vi "SetDevice_popup.vi"(2 "Input Line Command":string, 3 "error in (no error)":errorcluster) -> (8 "Cancel":bool, 9 "Output Line Command":string, 10 "error out":errorcluster)   [LabVIEW 2020]
uses:
  Device_List.ctl
  Unit_List.ctl
panel:
  in  "Motor":T1 caption="Unit"
  in  "platform":u16(ring) items=["Mac", "PC"]
  in  "372 unit":T1 caption="Unit"
  in  "372 ch#":T1 caption="Unit"
  in  "370 heater":T1 caption="Unit"
  in  "37X range":T1 caption="Unit"
  in  "37X Iex":T1 caption="Unit"
  in  "370 ch#":T1 caption="Unit"
  out "comment":string
  in  "heater value":T1 caption="Unit"
  in  "sensor value":T1 caption="Unit"
  in  "Cancel Button":bool
  in  "OK Button":bool
  in  "VISA resource name":refnum<visa-resource-name>
  in  "Unit":T1
  in  "Value":string="0"
  in  "Device":T2
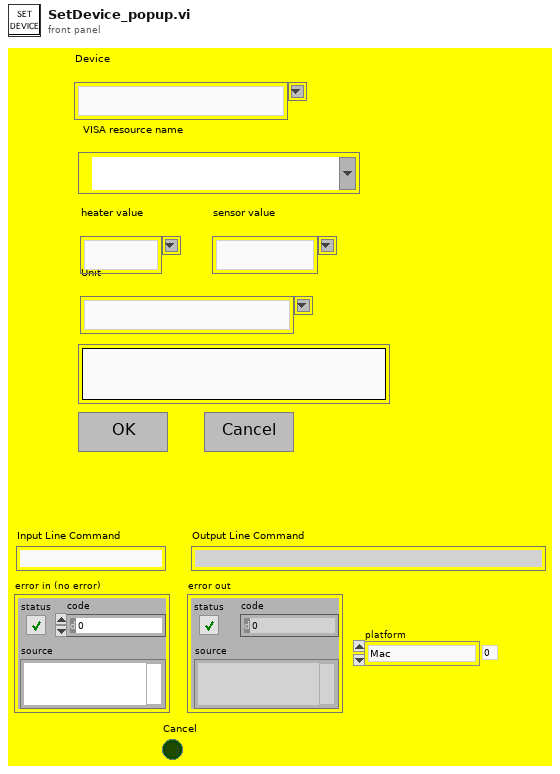
[diagram p1: front panel]
types:
  T1 = typedef "Unit_List.ctl" = string
  T2 = typedef "Device_List.ctl" = string
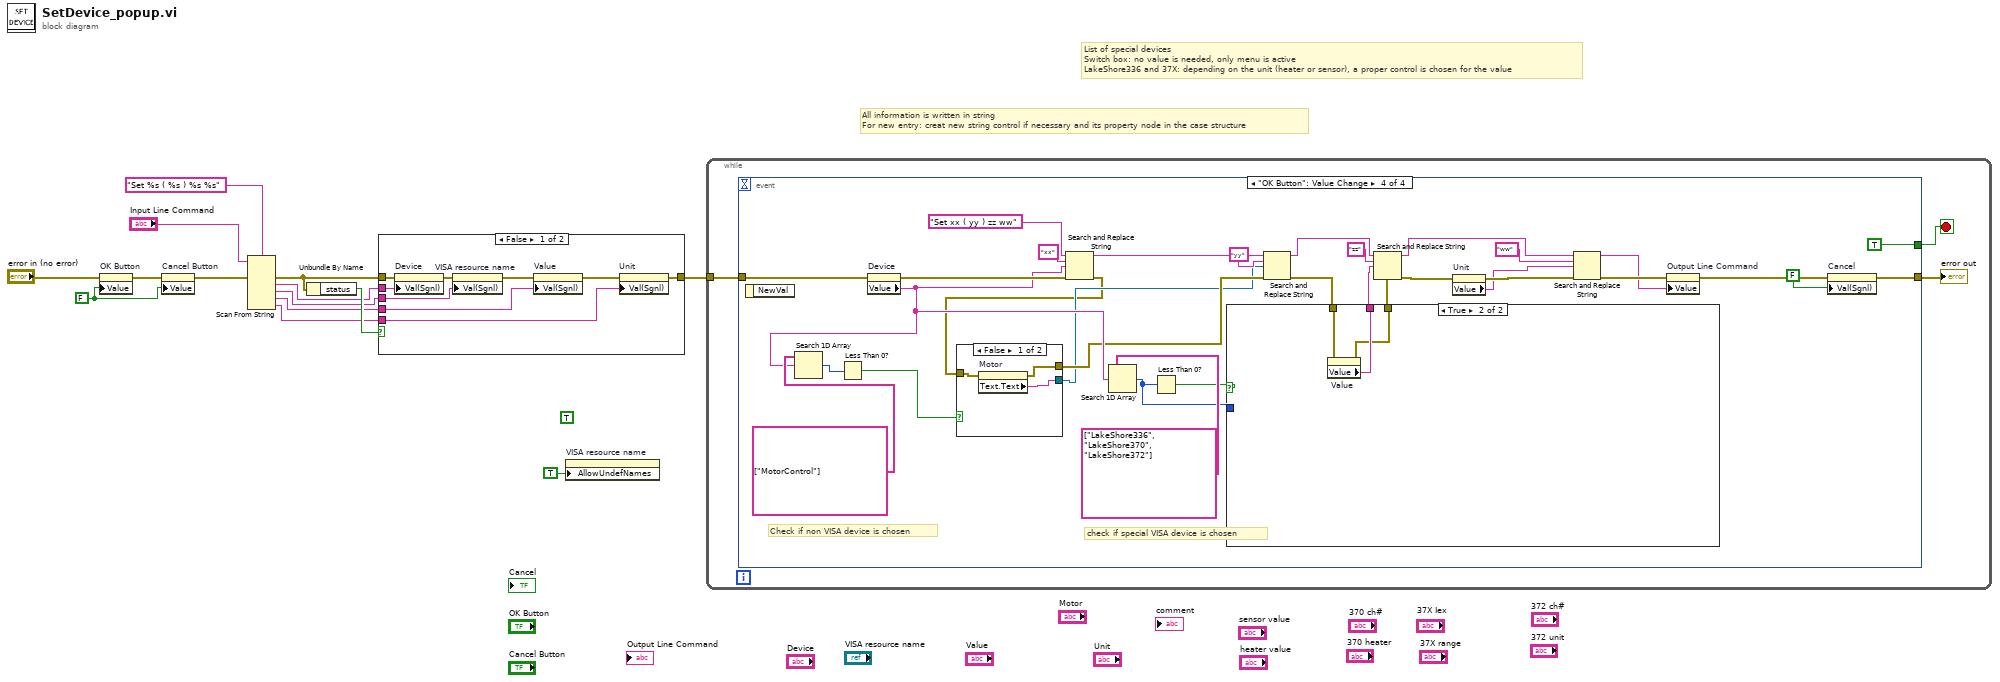
[diagram p0: block diagram]
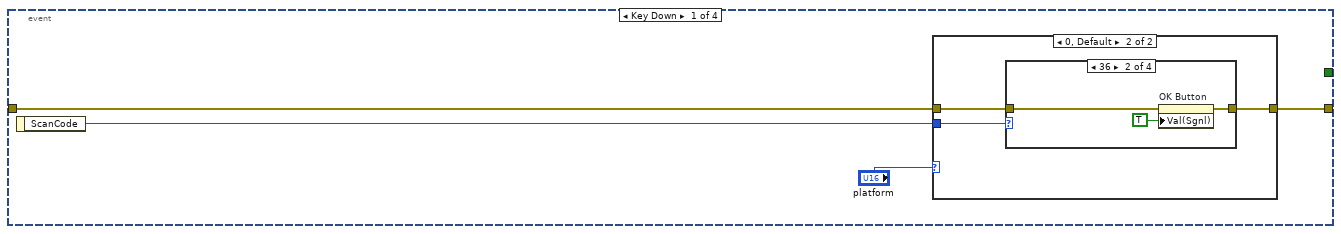
[diagram p2: hidden frame]
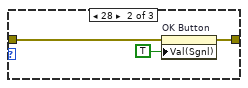
[diagram p4: hidden frame]
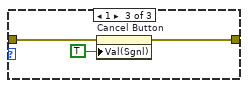
[diagram p5: hidden frame]
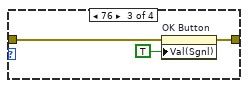
[diagram p7: hidden frame]
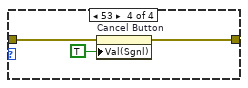
[diagram p8: hidden frame]
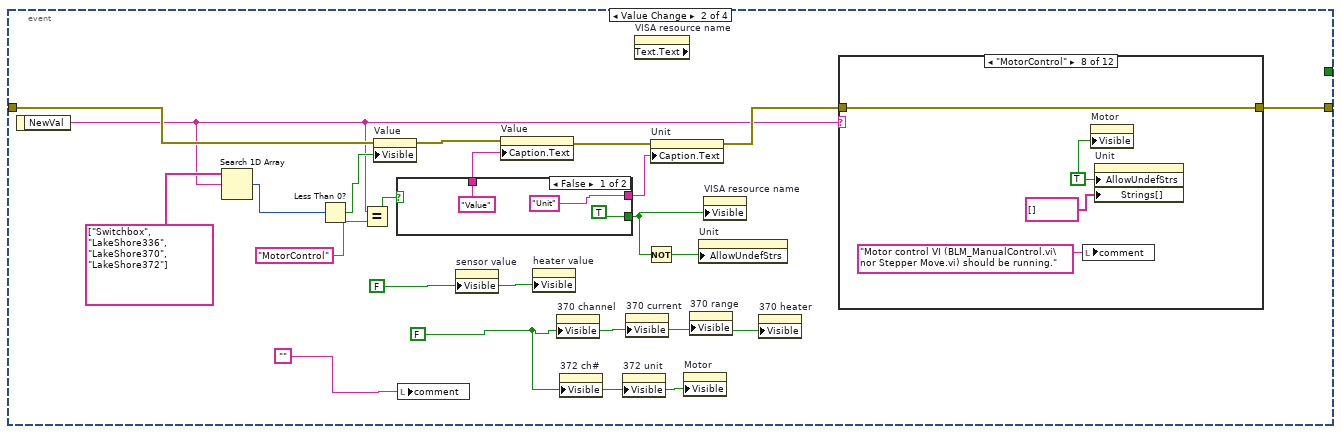
[diagram p9: hidden frame]
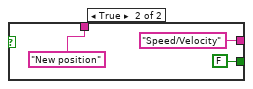
[diagram p10: hidden frame]
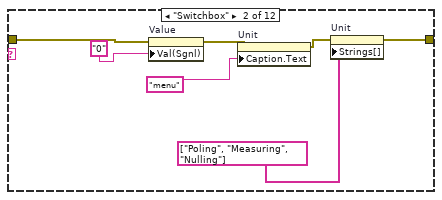
[diagram p12: hidden frame]
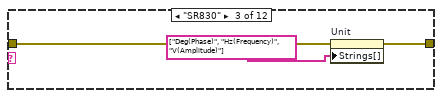
[diagram p13: hidden frame]
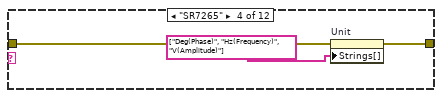
[diagram p14: hidden frame]
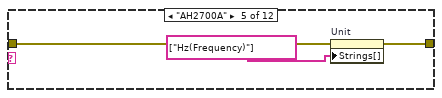
[diagram p15: hidden frame]
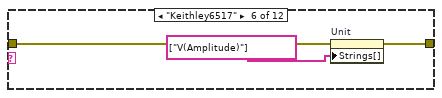
[diagram p16: hidden frame]
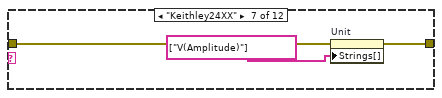
[diagram p17: hidden frame]
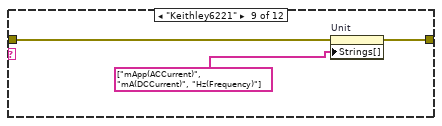
[diagram p18: hidden frame]
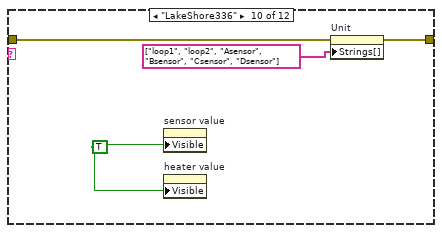
[diagram p19: hidden frame]
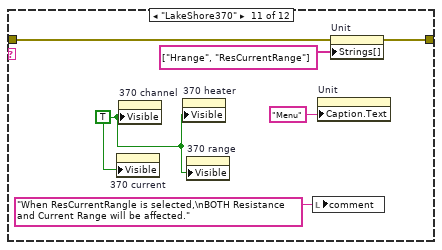
[diagram p20: hidden frame]
diagram:
  (unwired) TRUE ("Visible")
  w12 = FALSE
  # "List of special devices\nSwitch box: no value is needed, only menu is active\nLakeShore336 and 37X: depending on the unit (heater or sensor), a proper control is chosen for the value"
  # "All information is written in string\nFor new entry: creat new string control if necessary and its property node in the case structure"
  n1 = property on="OK Button" class="Bool (strict)"(error in="error in (no error)", "Value"=w12) -> (error out=w13:errorcluster)  [unwired: 1 in, 1 out]
  n2 = property on="Cancel Button" class="Bool (strict)"(error in=w13, "Value"=w12) -> (error out=w11:errorcluster)  [unwired: 1 in, 1 out]
  n3 = Scan From String(format string="Set %s ( %s ) %s %s", input string="Input Line Command", error in=w11) -> (error out=w7:errorcluster, output 1=w6:string, output 2=w5:string, output 3=w4:string, output 4=w3:string)  [unwired: 5 in, 2 out]
  n4 = Unbundle By Name(w7) -> ("status"=w8:bool)
  n5 = case shown="False" w8 {
    tunnel: w7 -> [w23 w25]
    tunnel: [w15 w24] -> w2
    tunnel: w6 -> [w22 _]
    tunnel: w5 -> [w20 _]
    tunnel: w4 -> [w18 _]
    tunnel: w3 -> [w16 _]
    frame False {
      n6 = property on="Device" class="CmbBox (strict)"(error in=w23, "Val(Sgnl)"=w22) -> (error out=w21:errorcluster)  [unwired: 1 in, 1 out]
      n7 = property on="VISA resource name" class="VISAName"(error in=w21, "Val(Sgnl)"=w20) -> (error out=w19:errorcluster)  [unwired: 1 in, 1 out]
      n8 = property on="Value" class="Str"(error in=w19, "Val(Sgnl)"=w18) -> (error out=w17:errorcluster)  [unwired: 1 in, 1 out]
      n9 = property on="Unit" class="CmbBox (strict)"(error in=w17, "Val(Sgnl)"=w16) -> (error out=w15:errorcluster)  [unwired: 1 in, 1 out]
    }
    frame True {
      n10 = call <vilib>:"Clear Errors.vi"("error in (no error)"=w25) -> ("error out"=w24:errorcluster)  [unwired: 5 in, 1 out]
    }
  }
  n11 = property on="VISA resource name" class="VISAName"("AllowUndefNames"=TRUE ("Allow Undefined Names")) -> ()  [unwired: 2 in, 2 out]
  n12 = while {
    tunnel: w2 -> [w28]
    stop <- w27 stop-if-true
    n13 = event shown="[3] \"OK Button\": Value Change" {
      selector: _ -> [_ _ _ _]
      dyn-events: _ -> [_ _ _ _]
      timeout: _ -> [_ _ _ _]
      tunnel: w28 -> [w31 w72 w127 w157]
      tunnel: [_ _ w126 TRUE ("NewVal")] -> w27
      tunnel: [w30 w73 _ w139] -> w26
      event Key Down {
        n14 = event-data() -> ("ScanCode"=w32:i16)  [unwired: 1 in]
        n15 = case shown="0, Default" "platform" {
          tunnel: w32 -> [w35 w45]
          tunnel: w31 -> [w34 w44]
          tunnel: [w33 w43] -> w30
          frame 1 {
            n16 = case shown="Default" w35 {
              tunnel: w34 -> [w36 w39 w42]
              tunnel: [w36 w37 w40] -> w33
              frame Default {
              }
              frame 28 {
                n17 = property on="OK Button" class="Bool (strict)"(error in=w39, "Val(Sgnl)"=TRUE) -> (error out=w37:errorcluster)  [unwired: 1 in, 1 out]
              }
              frame 1 {
                n18 = property on="Cancel Button" class="Bool (strict)"(error in=w42, "Val(Sgnl)"=TRUE ("Value (Signaling)")) -> (error out=w40:errorcluster)  [unwired: 1 in, 1 out]
              }
            }
          }
          frame 0, Default {
            n19 = case shown="36" w45 {
              tunnel: w44 -> [w46 w49 w52 w55]
              tunnel: [w46 w47 w50 w53] -> w43
              frame Default {
              }
              frame 36 {
                n20 = property on="OK Button" class="Bool (strict)"(error in=w49, "Val(Sgnl)"=TRUE) -> (error out=w47:errorcluster)  [unwired: 1 in, 1 out]
              }
              frame 76 {
                n21 = property on="OK Button" class="Bool (strict)"(error in=w52, "Val(Sgnl)"=TRUE) -> (error out=w50:errorcluster)  [unwired: 1 in, 1 out]
              }
              frame 53 {
                n22 = property on="Cancel Button" class="Bool (strict)"(error in=w55, "Val(Sgnl)"=TRUE ("Value (Signaling)")) -> (error out=w53:errorcluster)  [unwired: 1 in, 1 out]
              }
            }
          }
        }
      }
      event Value Change {
        w57 = FALSE ("Visible")
        w64 = FALSE ("Visible")
        n23 = event-data() -> ("NewVal"=w60:T2)  [unwired: 1 in]
        n24 = Search 1D Array(1D array=string[] ["Switchbox", "LakeShore336", "LakeShore370", "LakeShore372"], element=w60) -> (index of element=w70:i32)  [unwired: 1 in]
        n25 = Less Than 0?(x=w70) -> (x < 0?=w69:bool)
        n26 = Equal?(x=w60, y="MotorControl") -> (x = y?=w59:bool)
        n27 = property on="Value" class="Str"(error in=w72, "Visible"=w69) -> (error out=w67:errorcluster)  [unwired: 1 in, 1 out]
        n28 = case shown="False" w59 {
          tunnel: ["Value" ("Label.Text") "New position" ("Label.Text")] -> w68
          tunnel: ["Unit" ("Label.Text") "Speed/Velocity" ("Label.Text")] -> w62
          tunnel: [TRUE ("Visible") FALSE ("Visible")] -> w56
          frame False {
          }
          frame True {
          }
        }
        n29 = local write "comment"("") -> ()
        n30 = property on="sensor value" class="CmbBox (strict)"("Visible"=w64) -> ()  [unwired: 2 in, 2 out]
        n31 = property on="Value" class="Str"(error in=w67, "Caption.Text"=w68) -> (error out=w66:errorcluster)  [unwired: 1 in, 1 out]
        n32 = property on="heater value" class="CmbBox (strict)"("Visible"=w64) -> ()  [unwired: 2 in, 2 out]
        n33 = property on="370 channel" class="CmbBox (strict)"("Visible"=w57) -> ()  [unwired: 2 in, 2 out]
        n34 = property on="372 ch#" class="CmbBox (strict)"("Visible"=w57) -> ()  [unwired: 2 in, 2 out]
        n35 = property on="372 unit" class="CmbBox (strict)"("Visible"=w57) -> ()  [unwired: 2 in, 2 out]
        n36 = property on="370 current" class="CmbBox (strict)"("Visible"=w57) -> ()  [unwired: 2 in, 2 out]
        n37 = property on="VISA resource name" class="VISAName" props=["Text", "Text"]() -> ()  [unwired: 2 in, 3 out]
        n38 = Not(x=w56) -> (.not. x?=w58:bool)
        n39 = property on="Unit" class="CmbBox (strict)"(error in=w66, "Caption.Text"=w62) -> (error out=w65:errorcluster)  [unwired: 1 in, 1 out]
        n40 = property on="Motor" class="CmbBox (strict)"("Visible"=w57) -> ()  [unwired: 2 in, 2 out]
        n41 = property on="370 range" class="CmbBox (strict)"("Visible"=w57) -> ()  [unwired: 2 in, 2 out]
        n42 = property on="Unit" class="CmbBox (strict)"("AllowUndefStrs"=w58) -> ()  [unwired: 2 in, 2 out]
        n43 = property on="VISA resource name" class="VISAName"("Visible"=w56) -> ()  [unwired: 2 in, 2 out]
        n44 = property on="370 heater" class="CmbBox (strict)"("Visible"=w57) -> ()  [unwired: 2 in, 2 out]
        n45 = case shown="\"MotorControl\"" w60 {
          tunnel: w65 -> [w80 w87 w88 w91 w94 w97 w100 w106 w107 w111 w118 w124]
          tunnel: [w80 w85 w90 w93 w96 w99 w102 w106 w109 w113 w119 w125] -> w73
          frame "False", Default {
          }
          frame "Switchbox" {
            n46 = property on="Value" class="Str"(error in=w87, "Val(Sgnl)"="0" ("Value (Signaling)")) -> (error out=w83:errorcluster)  [unwired: 1 in, 1 out]
            n47 = property on="Unit" class="CmbBox (strict)"(error in=w83, "Caption.Text"="menu") -> (error out=w82:errorcluster)  [unwired: 1 in, 1 out]
            n48 = property on="Unit" class="CmbBox (strict)"(error in=w82, "Strings[]"=string[] ["Poling", "Measuring", "Nulling"] ("Strings []")) -> (error out=w85:errorcluster)  [unwired: 1 in, 1 out]
          }
          frame "SR830" {
            n49 = property on="Unit" class="CmbBox (strict)"(error in=w88, "Strings[]"=string[] ["Deg(Phase)", "Hz(Frequency)", "V(Amplitude)"] ("Strings []")) -> (error out=w90:errorcluster)  [unwired: 1 in, 1 out]
          }
          frame "SR7265" {
            n50 = property on="Unit" class="CmbBox (strict)"(error in=w91, "Strings[]"=string[] ["Deg(Phase)", "Hz(Frequency)", "V(Amplitude)"] ("Strings []")) -> (error out=w93:errorcluster)  [unwired: 1 in, 1 out]
          }
          frame "AH2700A" {
            n51 = property on="Unit" class="CmbBox (strict)"(error in=w94, "Strings[]"=string[] ["Hz(Frequency)"] ("Strings []")) -> (error out=w96:errorcluster)  [unwired: 1 in, 1 out]
          }
          frame "Keithley6517" {
            n52 = property on="Unit" class="CmbBox (strict)"(error in=w97, "Strings[]"=string[] ["V(Amplitude)"] ("Strings []")) -> (error out=w99:errorcluster)  [unwired: 1 in, 1 out]
          }
          frame "Keithley24XX" {
            n53 = property on="Unit" class="CmbBox (strict)"(error in=w100, "Strings[]"=string[] ["V(Amplitude)"] ("Strings []")) -> (error out=w102:errorcluster)  [unwired: 1 in, 1 out]
          }
          frame "MotorControl" {
            w103 = TRUE ("Allow Undefined Strings")
            n54 = local write "comment"("Motor control VI (BLM_ManualControl.vi\nor Stepper Move.vi) should be running." ("comment")) -> ()
            n55 = property on="Motor" class="CmbBox (strict)"("Visible"=w103) -> ()  [unwired: 2 in, 2 out]
            n56 = property on="Unit" class="CmbBox (strict)"("AllowUndefStrs"=w103, "Strings[]"=string[] [] ("Strings []")) -> ()  [unwired: 2 in, 2 out]
          }
          frame "Keithley6221" {
            n57 = property on="Unit" class="CmbBox (strict)"(error in=w107, "Strings[]"=string[] ["mApp(ACCurrent)", "mA(DCCurrent)", "Hz(Frequency)"] ("Strings []")) -> (error out=w109:errorcluster)  [unwired: 1 in, 1 out]
          }
          frame "LakeShore336" {
            w110 = TRUE ("Visible")
            n58 = property on="sensor value" class="CmbBox (strict)"("Visible"=w110) -> ()  [unwired: 2 in, 2 out]
            n59 = property on="heater value" class="CmbBox (strict)"("Visible"=w110) -> ()  [unwired: 2 in, 2 out]
            n60 = property on="Unit" class="CmbBox (strict)"(error in=w111, "Strings[]"=string[] ["loop1", "loop2", "Asensor", "Bsensor", "Csensor", "Dsensor"] ("Strings []")) -> (error out=w113:errorcluster)  [unwired: 1 in, 1 out]
          }
          frame "LakeShore370" {
            w116 = TRUE ("Visible")
            n61 = property on="370 current" class="CmbBox (strict)"("Visible"=w116) -> ()  [unwired: 2 in, 2 out]
            n62 = property on="370 channel" class="CmbBox (strict)"("Visible"=w116) -> ()  [unwired: 2 in, 2 out]
            n63 = property on="370 heater" class="CmbBox (strict)"("Visible"=w116) -> ()  [unwired: 2 in, 2 out]
            n64 = property on="370 range" class="CmbBox (strict)"("Visible"=w116) -> ()  [unwired: 2 in, 2 out]
            n65 = local write "comment"("When ResCurrentRangle is selected,\nBOTH Resistance and Current Range will be affected." ("comment")) -> ()
            n66 = property on="Unit" class="CmbBox (strict)"("Caption.Text"="Menu") -> ()  [unwired: 2 in, 2 out]
            n67 = property on="Unit" class="CmbBox (strict)"(error in=w118, "Strings[]"=string[] ["Hrange", "ResCurrentRange"] ("Strings []")) -> (error out=w119:errorcluster)  [unwired: 1 in, 1 out]
          }
          frame "LakeShore372" {
            w120 = TRUE ("Visible")
            n68 = property on="370 current" class="CmbBox (strict)"("Visible"=w120) -> ()  [unwired: 2 in, 2 out]
            n69 = property on="372 ch#" class="CmbBox (strict)"("Visible"=w120) -> ()  [unwired: 2 in, 2 out]
            n70 = property on="370 range" class="CmbBox (strict)"("Visible"=w120) -> ()  [unwired: 2 in, 2 out]
            n71 = property on="372 unit" class="CmbBox (strict)"("Visible"=w120) -> ()  [unwired: 2 in, 2 out]
            n72 = property on="Unit" class="CmbBox (strict)"("Caption.Text"="Menu") -> ()  [unwired: 2 in, 2 out]
            n73 = property on="Unit" class="CmbBox (strict)"(error in=w124, "Strings[]"=string[] ["ResCurrentRange"] ("Strings []")) -> (error out=w125:errorcluster)  [unwired: 1 in, 1 out]
            n74 = local write "comment"("When ResCurrentRangle is selected,\nAll parameters (Resistance, Current Range, unit) will be affected." ("comment")) -> ()
          }
        }
      }
      event "Cancel Button": Value Change {
        n75 = event-data() -> ("NewVal"=w126:bool)  [unwired: 1 in]
        n76 = property on="Cancel" class="Bool (strict)"(error in=w127, "Value"=w126) -> ()  [unwired: 1 in, 2 out]
      }
      event "OK Button": Value Change {
        # "Check if non VISA device is chosen"
        # "check if special VISA device is chosen"
        n77 = event-data() -> ()  [unwired: 1 in, 1 out]
        n78 = property on="Device" class="CmbBox (strict)"(error in=w157) -> (error out=w156:errorcluster, "Value"=w131:T2)  [unwired: 1 in, 1 out]
        n79 = Search 1D Array(1D array=string[] ["MotorControl"], element=w131) -> (index of element=w134:i32)  [unwired: 1 in]
        n80 = Less Than 0?(x=w134) -> (x < 0?=w133:bool)
        n81 = Search and Replace String(input string="Set xx ( yy ) zz ww", search string="xx", replace string=w131, error in=w156) -> (result string=w154:string, error out=w128:errorcluster)  [unwired: 4 in, 2 out]
        n82 = case shown="False" w133 {
          tunnel: [w161 w165] -> w130
          tunnel: [w160 w164] -> w129
          tunnel: w128 -> [w162 w163]
          frame False {
            n83 = property on="Motor" class="CmbBox (strict)"(error in=w162) -> (error out=w161:errorcluster, "Text.Text"=w160:string)  [unwired: 1 in, 1 out]
          }
          frame True {
            n84 = property on="VISA resource name" class="VISAName"(error in=w163) -> (error out=w165:errorcluster, "Value"=w164:refnum<visa-resource-name>)  [unwired: 1 in, 1 out]
          }
        }
        n85 = Search 1D Array(1D array=string[] ["LakeShore336", "LakeShore370", "LakeShore372"], element=w131) -> (index of element=w135:i32)  [unwired: 1 in]
        n86 = Less Than 0?(x=w135) -> (x < 0?=w136:bool)
        n87 = Search and Replace String(input string=w154, search string="yy", replace string=w129, error in=w130) -> (result string=w153:string, error out=w150:errorcluster)  [unwired: 4 in, 2 out]
        n88 = case shown="True" w136 {
          tunnel: [w166 w222] -> w151
          tunnel: w150 -> [w168 w221]
          tunnel: [w167 w220] -> w149
          tunnel: w135 -> [w169 _]
          frame False {
            n89 = case shown="1" w169 {
              tunnel: w168 -> [w174 w190 w208]
              tunnel: [w173 w189 w207] -> w167
              tunnel: [w172 w184 w203] -> w166
              frame 0, Default {
                # "Lakeshore336"
                n90 = property on="Unit" class="CmbBox (strict)"() -> ("Text.Text"=w170:string)  [unwired: 2 in, 2 out]
                n91 = Match Pattern(string=w170, regular expression="loop") -> (offset past match=w175:i32)  [unwired: 1 in, 3 out]
                n92 = Less Than 0?(x=w175) -> (x < 0?=w171:bool)
                n93 = case shown="False" w171 {
                  tunnel: w174 -> [w179 w182]
                  tunnel: [w178 w181] -> w173
                  tunnel: [w177 w180] -> w172
                  frame False {
                    n94 = property on="heater value" class="CmbBox (strict)"(error in=w179) -> (error out=w178:errorcluster, "Text.Text"=w177:string)  [unwired: 1 in, 1 out]
                  }
                  frame True {
                    n95 = property on="sensor value" class="CmbBox (strict)"(error in=w182) -> (error out=w181:errorcluster, "Text.Text"=w180:string)  [unwired: 1 in, 1 out]
                  }
                }
              }
              frame 1 {
                # "Lakeshore336"
                n96 = property on="Unit" class="CmbBox (strict)"() -> ("Text.Text"=w188:string)  [unwired: 2 in, 2 out]
                n97 = property on="370 channel" class="CmbBox (strict)"() -> ("Text.Text"=w186:string)  [unwired: 2 in, 2 out]
                n98 = case shown="\"ResCurrentRange\"" w188 {
                  tunnel: w190 -> [w193 w197]
                  tunnel: [w192 w195] -> w189
                  tunnel: [w191 w198] -> w183
                  frame "Hrange", Default {
                    n99 = property on="370 heater" class="CmbBox (strict)"(error in=w193) -> (error out=w192:errorcluster, "Text.Text"=w191:string)  [unwired: 1 in, 1 out]
                  }
                  frame "ResCurrentRange" {
                    n100 = property on="370 Iex" class="CmbBox (strict)"(error in=w197) -> (error out=w196:errorcluster, "Text.Text"=w194:string)  [unwired: 1 in, 1 out]
                    n101 = property on="370 range" class="CmbBox (strict)"(error in=w196) -> (error out=w195:errorcluster, "Text.Text"=w199:string)  [unwired: 1 in, 1 out]
                    n102 = Concatenate Strings(w194, "::" ("string"), w199) -> (w198:string)
                  }
                }
                n103 = Concatenate Strings("Channel_" ("string"), w186, "::" ("string"), w183) -> (w184:string)
              }
              frame 2 {
                # "Lakeshore336"
                n104 = property on="Unit" class="CmbBox (strict)"() -> ("Text.Text"=w206:string)  [unwired: 2 in, 2 out]
                n105 = property on="372 ch#" class="CmbBox (strict)"() -> ("Text.Text"=w201:string)  [unwired: 2 in, 2 out]
                n106 = case shown="\"ResCurrentRange\"" w206 {
                  tunnel: w208 -> [w211 w217]
                  tunnel: [w210 w215] -> w207
                  tunnel: [w209 w218] -> w202
                  frame "Hrange", Default {
                    n107 = property on="370 heater" class="CmbBox (strict)"(error in=w211) -> (error out=w210:errorcluster, "Text.Text"=w209:string)  [unwired: 1 in, 1 out]
                  }
                  frame "ResCurrentRange" {
                    w213 = "::" ("string")
                    n108 = property on="372 unit" class="CmbBox (strict)"() -> ("Text.Text"=w212:string)  [unwired: 2 in, 2 out]
                    n109 = property on="370 Iex" class="CmbBox (strict)"(error in=w217) -> (error out=w216:errorcluster, "Text.Text"=w214:string)  [unwired: 1 in, 1 out]
                    n110 = property on="370 range" class="CmbBox (strict)"(error in=w216) -> (error out=w215:errorcluster, "Text.Text"=w219:string)  [unwired: 1 in, 1 out]
                    n111 = Concatenate Strings(w214, w213, w219, w213, w212) -> (w218:string)
                  }
                }
                n112 = Concatenate Strings("Channel_" ("string"), w201, "::" ("string"), w202) -> (w203:string)
              }
            }
          }
          frame True {
            n113 = property on="Value" class="Str"(error in=w221) -> (error out=w220:errorcluster, "Value"=w222:string)  [unwired: 1 in, 1 out]
          }
        }
        n114 = Search and Replace String(input string=w153, search string="zz", replace string=w151, error in=w149) -> (result string=w148:string, error out=w147:errorcluster)  [unwired: 4 in, 2 out]
        n115 = property on="Unit" class="CmbBox (strict)"(error in=w147) -> (error out=w146:errorcluster, "Value"=w145:T1)  [unwired: 1 in, 1 out]
        n116 = Search and Replace String(input string=w148, search string="ww", replace string=w145, error in=w146) -> (result string=w142:string, error out=w143:errorcluster)  [unwired: 4 in, 2 out]
        n117 = property on="Output Line Command" class="Str"(error in=w143, "Value"=w142) -> (error out=w141:errorcluster)  [unwired: 1 in, 1 out]
        n118 = property on="Cancel" class="Bool (strict)"(error in=w141, "Val(Sgnl)"=FALSE ("Cancel")) -> (error out=w139:errorcluster)  [unwired: 1 in, 1 out]
      }
    }
    "error out" <- w26
  }
